vi "Fail.vi"(7 "Caller":string, 8 "error in (no error)":errorcluster, 9 "Message":string, 10 "Assertion":string) -> (0 "error out":errorcluster)   [LabVIEW 2017, in "Caraya Adapter.lvclass"]
uses:
  Caraya Adapter.lvclass
  <vilib>/addons/_JKI Toolkits/Caraya/classes/Properties.Assert/Properties.Assert.lvclass
  C:/Program Files/National Instruments/LabVIEW 2017/vi.lib/addons/_JKI Toolkits/Caraya/classes/Properties/Properties.lvclass
  <vilib>/addons/_JKI Toolkits/Caraya/classes/Assert/Assert.lvclass
  <vilib>/addons/_JKI Toolkits/Caraya/classes/Properties/Properties.lvclass
  Error/Error.lvlib
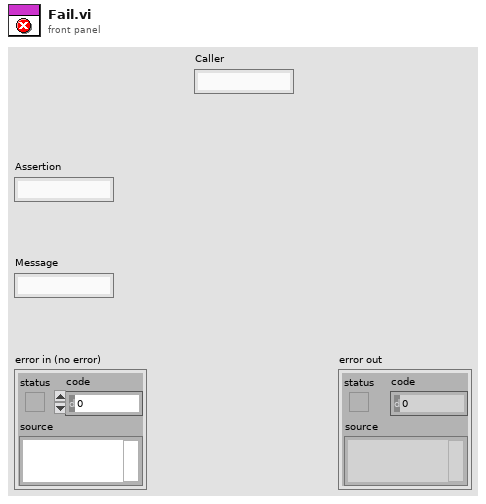
[diagram p1: front panel]
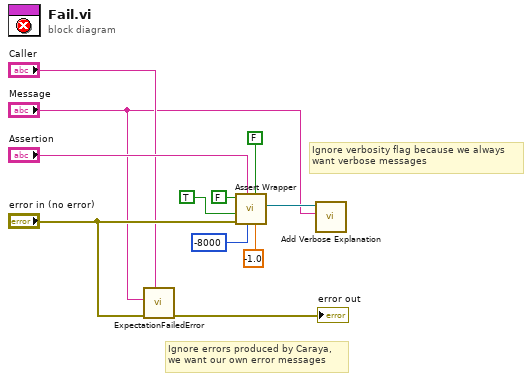
[diagram p0: block diagram]
diagram:
  # "Ignore errors produced by Caraya,\nwe want our own error messages"
  # "Ignore verbosity flag because we always\nwant verbose messages"
  n1 = call "ExpectationFailedError.vi"("Source (caller)"="Caller", "error in (no error)"="error in (no error)", "Message"="Message") -> ("error out"=→"error out":errorcluster)  [unwired: 8 in]
  n2 = call <vilib>:"Assert Wrapper.vi"("Execution time (s)"=-1.0, "Assert Only? (F)"=FALSE, "error code (1)"=-8000, "Label"="Assertion", "error in (no error)"="error in (no error)", "Register with caller test (F)"=TRUE, "Assert?"=FALSE) -> ("Properties.Assert"=w6:refnum<class "Properties.Assert.lvclass">)  [unwired: 1 in, 3 out]
  n3 = call <vilib>:"Add Verbose Explanation.vi"("Verbose Explanation"="Message", "Properties"=w6) -> ()  [unwired: 8 in, 2 out]
